vi "按钮旋转sin.vi"() -> ()   [LabVIEW 2018]
panel:
  in  "确定按钮":bool
  out "布尔":bool
  in  "停止":bool
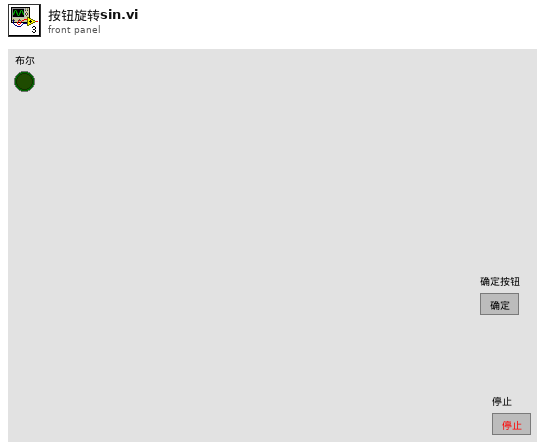
[diagram p1: front panel]
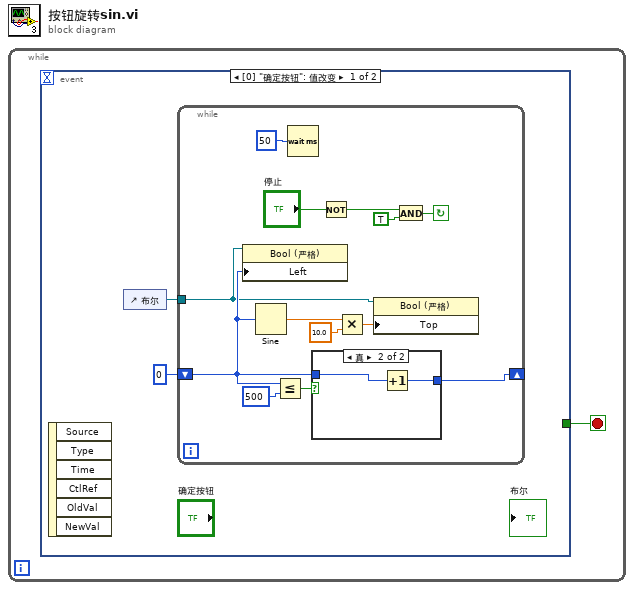
[diagram p0: block diagram]
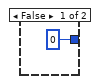
[diagram p2: hidden frame]
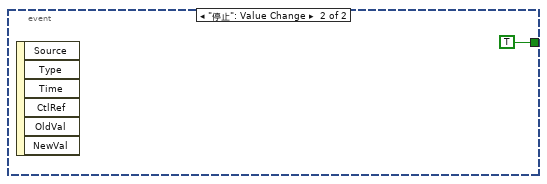
[diagram p3: hidden frame]
diagram:
  n1 = while {
    stop <- w1 stop-if-true
    n2 = event shown="[0] \"确定按钮\": 值改变" {
      selector: _ -> [_ _]
      dyn-events: _ -> [_ _]
      timeout: _ -> [_ _]
      tunnel: [_ TRUE] -> w1
      event "确定按钮": Value Change {
        n3 = event-data() -> ()  [unwired: 1 in, 6 out]
        n4 = control-ref of="布尔"() -> (w2:refnum<vi>)
        n5 = while {
          shift-right: [w14] -> _
          shift-left: 0 -> [w13]
          tunnel: w2 -> [w4]
          stop <- w6 continue-if-true
          n6 = property on="属性节点" class="Bool (严格)"(reference=w4, "Left"=w13) -> ()  [unwired: 1 in, 2 out]
          n7 = Sine(x=w13) -> (sin(x)=w11:dbl)
          n8 = Less Or Equal?(x=w13, y=500) -> (x <= y?=w16:bool)
          n9 = Wait (ms)(milliseconds to wait=u32 50 ("等待时间（毫秒）")) -> ()  [unwired: 1 out]
          n10 = case shown="真" w16 {
            tunnel: w13 -> [_ w19]
            tunnel: [0 w18] -> w14
            frame False {
            }
            frame True {
              n11 = Increment(x=w19) -> (x+1=w18:i32)
            }
          }
          n12 = Not(x="停止") -> (.not. x?=w7:bool)
          n13 = Multiply(x=w11, y=10.0) -> (x*y=w10:dbl)
          n14 = property on="属性节点" class="Bool (严格)"(reference=w4, "Top"=w10) -> ()  [unwired: 1 in, 2 out]
          n15 = And(x=w7, y=TRUE) -> (x .and. y?=w6:bool)
        }
      }
      event "停止": Value Change {
        n16 = event-data() -> ()  [unwired: 1 in, 6 out]
      }
    }
  }
